vi "Actor Core.vi"(8 "error in":errorcluster, 11 "Example Actor in":refnum<class "Example Actor.lvclass">) -> (0 "error out":errorcluster, 3 "Actor out":refnum<class "Actor.lvclass">)   [LabVIEW 2023, in "Example Iterator NR Actor.lvlib" / "Example Actor.lvclass"]
doc: "(<B>Filename</B>: Actor Framework.lvlib:Actor.lvclass:Actor Core.vi)\n\nReceives messages to the actor, reacts to them, and initiates any error handling that may shut the actor down.\n\nDescendant classes may override this VI to append parallel tasks for the actor to complete while it handles messages. Overrides use the Call Parent Method node."
uses:
  Example Actor.lvclass
  C:/Program Files/National Instruments/LabVIEW 2023/vi.lib/ActorFramework/Actor/Actor.lvclass
  <vilib>/ActorFramework/Actor/Actor.lvclass
  Iterator Settings.ctl
  Abstract Iterator Actor/Active Stop Conditions.ctl
  <vilib>/ActorFramework/Message Enqueuer/Message Priority.ctl
  Abstract Iterator Actor/Stop Reason.ctl
  Iterator NR Actor/Iterator NR Actor.lvclass
  Iterator NR Actor/Iterator NR Actor.lvclass/Iterator NR Actor.ctl
  Example Actor.lvclass/Example Actor.ctl
  <vilib>/ActorFramework/Actor/Actor.lvclass/Actor.ctl
  <vilib>/ActorFramework/Message Enqueuer/Message Enqueuer.lvclass/Message Enqueuer.ctl
  Example Actor Messages/Iterate Reply Msg/Iteration Msg.lvclass
  C:/Program Files/National Instruments/LabVIEW 2023/vi.lib/ActorFramework/Message/Message.lvclass
  Abstract Iterator Actor/Iterator Settings.ctl
  <vilib>/ActorFramework/Message/Message.lvclass
  Abstract Iterator Actor Messages/Iterator Report Iterations End Msg/Iterator Report Iterations End Msg.lvclass
  Example Actor Messages/Pre Iterate Reply Msg/Pre Iteration Msg.lvclass
  Example Actor Messages/Post Iterate Reply Msg/Post Iteration Msg.lvclass
  Example Actor Messages/Update Error Msg/Update Error Msg.lvclass
  C:/Projects/Iterator Actor/Abstract Iterator Actor Messages/Iterator Report Iterations End Msg/Iterator Report Iterations End Msg.lvclass
  Iterator NR Actor/Write Auto Iteration Notification.vi
  <vilib>/ActorFramework/Message Enqueuer/Init from Existing Queue.vi
  <vilib>/ActorFramework/Message Enqueuer/Enqueue.vi
  <vilib>/ActorFramework/Stop Msg/Stop Msg.lvclass
  <vilib>/ActorFramework/Message Priority Queue/Priority Enqueue.vi
  <vilib>/ActorFramework/Message Enqueuer/Message Enqueuer.lvclass
  Abstract Iterator Actor Messages/Write Settings Msg/Write Settings Msg.lvclass
  Abstract Iterator Actor Messages/Start Iterations Msg/Start Iterations Msg.lvclass
  Abstract Iterator Actor Messages/Stop Iterations Msg/Stop Iterations Msg.lvclass
  Abstract Iterator Actor/Abstract Iterator Actor.lvclass
panel:
  out "Stop Reason":T1
  in  "Receive report":bool=TRUE
  in  "Do post-iterations":bool=TRUE
  in  "Do pre-iterations":bool=TRUE
  out "Iterator error":errorcluster
  in  "User Settings":T2={"Prepare timeout (ms)"=1000, "Iterate timeout (ms)"=1000, "Conclude timeout (ms)"=1000, "Iterate period (ms)"=1000, "Active Stop Conditions"={"Number of Iterations"=FALSE, "Time Elapsed"=FALSE, "Iteration Result"=FALSE}, "Iterations"=5, "Time before stop (ms)"=200, "Message Priority (Normal)"=enum."Normal"}
  out "Post Iterate":bool
  out "Pre Iterate":bool
  in  "exit":bool
  out "Iterate":bool
  in  "stop iterations":bool
  in  "start iterations":bool
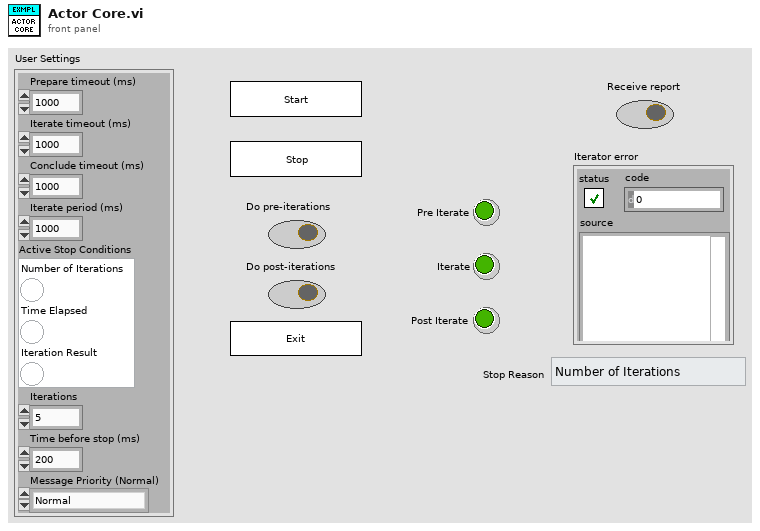
[diagram p1: front panel]
types:
  T1 = typedef "Iterator Actor.lvlib/Abstract Iterator Actor.lvclass/Stop Reason.ctl" = enum16{"Number of Iterations", "Time Elapsed", "Stopped Internally", "Stopped Externally"}
  T2 = typedef "Example Iterator NR Actor.lvlib/Example Actor.lvclass/Iterator Settings.ctl" = cluster{"Prepare timeout (ms)":i32, "Iterate timeout (ms)":i32, "Conclude timeout (ms)":i32, "Iterate period (ms)":i32, "Active Stop Conditions":T3, "Iterations":i32, "Time before stop (ms)":i32, "Message Priority (Normal)":T4}
  T3 = typedef "Iterator Actor.lvlib/Abstract Iterator Actor.lvclass/Active Stop Conditions.ctl" = cluster{"Number of Iterations":bool, "Time Elapsed":bool, "Iteration Result":bool}
  T4 = typedef "Actor Framework.lvlib/Message Enqueuer.lvclass/Message Priority.ctl" = enum16{"Low", "Normal", "High"}
  T5 = typedef "Iterator Actor.lvlib/Abstract Iterator Actor.lvclass/Iterator Settings.ctl" = cluster{"Prepare timeout (ms)":i32, "Iterate timeout (ms)":i32, "Conclude timeout (ms)":i32, "Iterate period (ms)":i32, "Number of iterations":i32, "Time before stop (ms)":i32, "Active Stop Conditions":T3, "Prepare Msg":refnum<class "Message.lvclass">, "Iterate Msg":refnum<class "Message.lvclass">, "Conclude Msg":refnum<class "Message.lvclass">, "Iterations End Report":refnum<class "Iterator Report Iterations End Msg.lvclass">, "Message Priority (Normal)":T4}
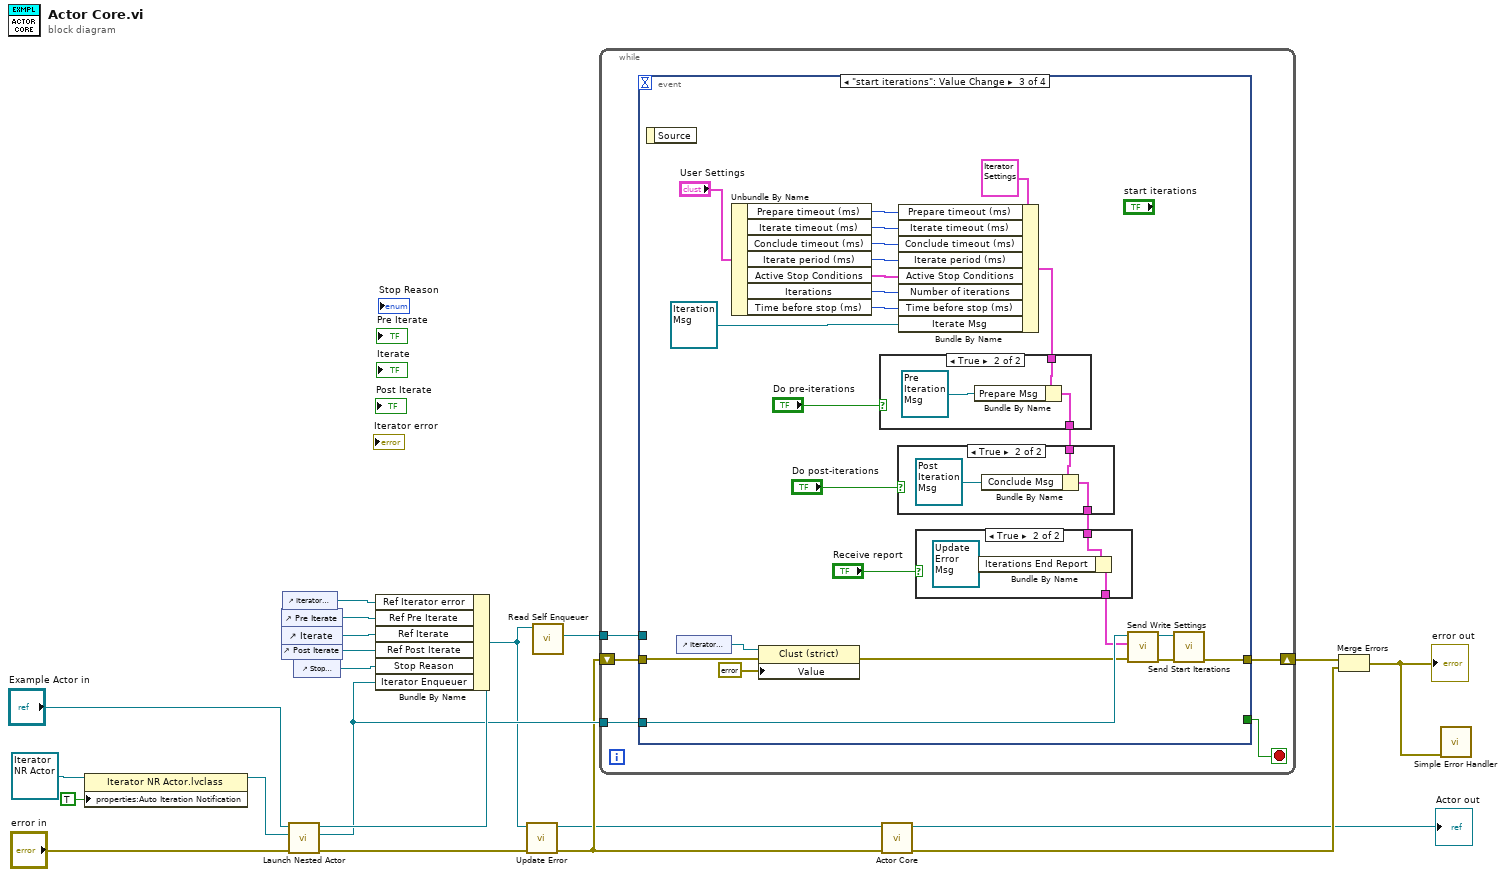
[diagram p0: block diagram]
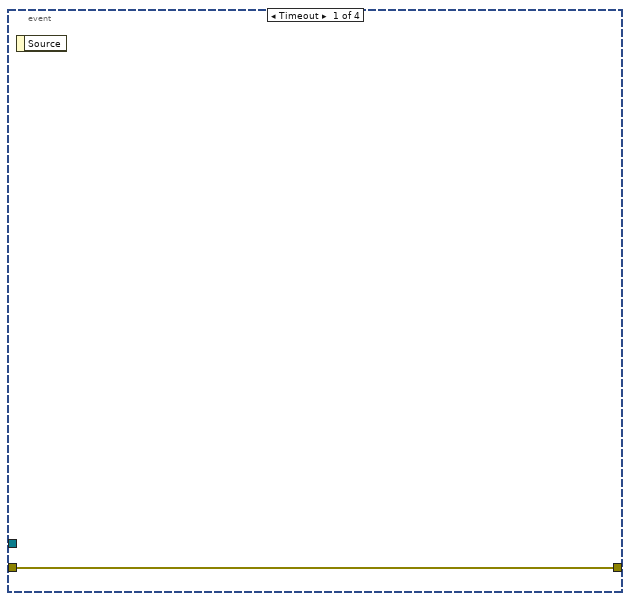
[diagram p2: hidden frame]
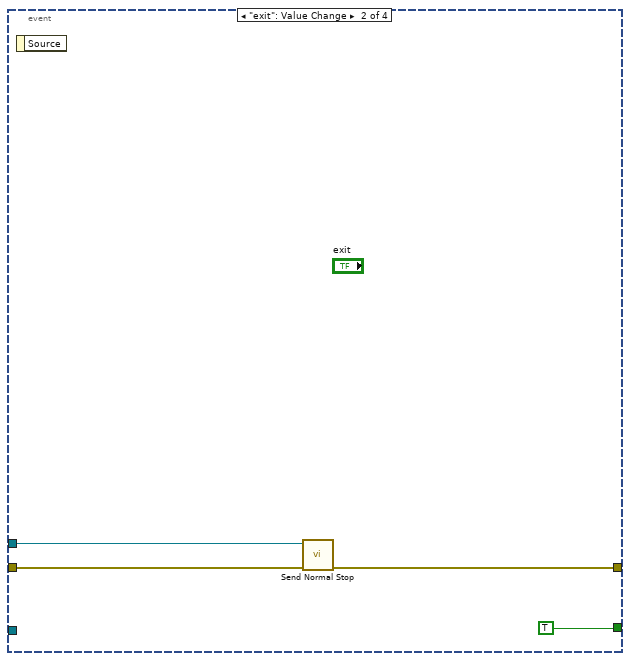
[diagram p3: hidden frame]
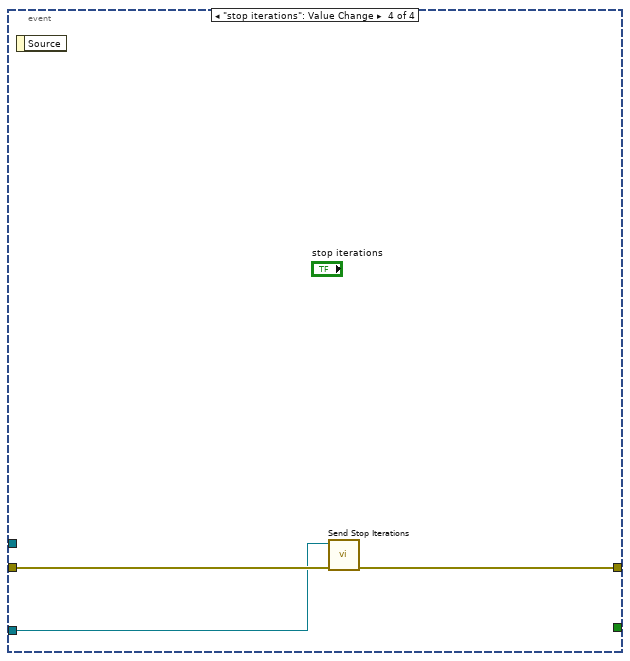
[diagram p7: hidden frame]
diagram:
  n1 = property class="Iterator NR Actor.lvclass"(reference=refnum<class "Iterator NR Actor.lvclass"> refnum ("Iterator Actor 2.lvlib:Iterator Actor 2.lvclass"), "properties:Auto Iteration Notification"=TRUE ("Auto Iteration Notification")) -> (reference out=w2:refnum<class "Iterator NR Actor.lvclass">)  [unwired: 1 in, 1 out]
  n2 = control-ref of="Pre Iterate"() -> (w17:refnum<vi>)
  n3 = control-ref of="Iterate"() -> (w16:refnum<vi>)
  n4 = control-ref of="Post Iterate"() -> (w15:refnum<vi>)
  n5 = control-ref of="Iterator error"() -> (w11:refnum<vi>)
  n6 = call <vilib>:"Launch Nested Actor.vi"("error in (no error)"="error in", "Nested Actor"=w2, "Caller Actor in"="Example Actor in") -> ("error out"=w10:errorcluster, "Nested Actor's Enqueuer"=w13:refnum<class "Message Enqueuer.lvclass">, "Caller Actor out"=w14:refnum<class "Example Actor.lvclass">)  [unwired: 6 in]
  n7 = control-ref of="Stop Reason"() -> (w6:refnum<vi>)
  n8 = Bundle By Name(cluster=w14, "Ref Iterator error"=w11, "Ref Pre Iterate"=w17, "Ref Iterate"=w16, "Ref Post Iterate"=w15, "Stop Reason"=w6, "Iterator Enqueuer"=w13) -> (w8:refnum<class "Example Actor.lvclass">)
  n9 = call "Update Error.vi"("error in (no error)"=w10, "Example Actor in"=w8) -> ("error out"=w9:errorcluster, "Example Actor out"=w7:refnum<class "Example Actor.lvclass">)  [unwired: 8 in]
  n10 = call <vilib>:"Read Self Enqueuer.vi"("Actor"=w8) -> ("Self Enqueuer"=w21:refnum<class "Message Enqueuer.lvclass">)  [unwired: 10 in]
  n11 = while {
    tunnel: w21 -> [w26]
    shift-right: [w25] -> w20
    shift-left: w9 -> [w24]
    tunnel: w13 -> [w22]
    stop <- w23 stop-if-true
    n12 = event shown="[2] \"start iterations\": Value Change" {
      selector: _ -> [_ _ _ _]
      dyn-events: _ -> [_ _ _ _]
      timeout: _ -> [_ _ _ _]
      tunnel: w26 -> [_ w31 _ _]
      tunnel: [w27 w30 w41 w70] -> w25
      tunnel: w24 -> [w27 w29 w44 w71]
      tunnel: [_ TRUE _ _] -> w23
      tunnel: w22 -> [_ _ w55 w69]
      event Timeout {
        n13 = event-data() -> ()  [unwired: 1 in, 1 out]
      }
      event "exit": Value Change {
        n14 = event-data() -> ()  [unwired: 1 in, 1 out]
        n15 = call <vilib>:"Send Normal Stop.vi"("error in (no error)"=w29, "Message Enqueuer"=w31) -> ("error out"=w30:errorcluster)  [unwired: 9 in]
      }
      event "start iterations": Value Change {
        n16 = event-data() -> ()  [unwired: 1 in, 1 out]
        n17 = control-ref of="Iterator error"() -> (w43:refnum<vi>)
        n18 = Unbundle By Name("User Settings") -> ("Prepare timeout (ms)"=w48:i32, "Iterate timeout (ms)"=w49:i32, "Conclude timeout (ms)"=w50:i32, "Iterate period (ms)"=w51:i32, "Active Stop Conditions"=w45:T3, "Iterations"=w46:i32, "Time before stop (ms)"=w47:i32)
        n19 = property class="Clust (strict)"(reference=w43, error in=w44, "Value"=errorcluster {"status"=FALSE, "code"=0, "source"=""}) -> (error out=w39:errorcluster)  [unwired: 1 out]
        n20 = Bundle By Name(cluster=T5 {"Prepare timeout (ms)"=0, "Iterate timeout (ms)"=0, "Conclude timeout (ms)"=0, "Iterate period (ms)"=0, "Number of iterations"=0, "Time before stop (ms)"=0, "Active Stop Conditions"={"Number of Iterations"=FALSE, "Time Elapsed"=FALSE, "Iteration Result"=FALSE}, "Prepare Msg"=refnum, "Iterate Msg"=refnum, "Conclude Msg"=refnum, "Iterations End Report"=refnum, "Message Priority (Normal)"=enum."Normal"} ("Iterator Settings"), "Prepare timeout (ms)"=w48, "Iterate timeout (ms)"=w49, "Conclude timeout (ms)"=w50, "Iterate period (ms)"=w51, "Active Stop Conditions"=w45, "Number of iterations"=w46, "Time before stop (ms)"=w47, "Iterate Msg"=refnum<class "Iteration Msg.lvclass"> refnum ("Example Actor.lvlib:Iterate Reply Msg.lvclass")) -> (w36:T5)
        n21 = case shown="True" "Do pre-iterations" {
          tunnel: w36 -> [w65 w68]
          tunnel: [w65 w66] -> w35
          frame False {
          }
          frame True {
            n22 = Bundle By Name(cluster=w68, "Prepare Msg"=refnum<class "Pre Iteration Msg.lvclass"> refnum ("Example Actor.lvlib:Pre Iterate Reply Msg.lvclass")) -> (w66:T5)
          }
        }
        n23 = case shown="True" "Do post-iterations" {
          tunnel: w35 -> [w61 w64]
          tunnel: [w61 w62] -> w33
          frame False {
          }
          frame True {
            n24 = Bundle By Name(cluster=w64, "Conclude Msg"=refnum<class "Post Iteration Msg.lvclass"> refnum ("Example Actor.lvlib:Post Iterate Reply Msg.lvclass")) -> (w62:T5)
          }
        }
        n25 = case shown="True" "Receive report" {
          tunnel: [w57 w60] -> w32
          tunnel: w33 -> [w57 w59]
          frame False {
          }
          frame True {
            n26 = Bundle By Name(cluster=w59, "Iterations End Report"=refnum<class "Update Error Msg.lvclass"> refnum ("Example Actor.lvlib:Update Error Msg.lvclass")) -> (w60:T5)
          }
        }
        n27 = call "Send Write Settings.vi"("error in (no error)"=w39, "Settings"=w32, "Message Enqueuer in"=w55) -> ("error out"=w56:errorcluster, "Message Enqueuer out"=w40:refnum<class "Message Enqueuer.lvclass">)  [unwired: 7 in]
        n28 = call "Send Start Iterations.vi"("error in (no error)"=w56, "Message Enqueuer in"=w40) -> ("error out"=w41:errorcluster)  [unwired: 8 in, 1 out]
      }
      event "stop iterations": Value Change {
        n29 = event-data() -> ()  [unwired: 1 in, 1 out]
        n30 = call "Send Stop Iterations.vi"("error in (no error)"=w71, "Message Enqueuer in"=w69) -> ("error out"=w70:errorcluster)  [unwired: 8 in, 1 out]
      }
    }
  }
  n31 = call-parent "Actor Core.vi"("error in"=w9, "Actor in"=w7) -> ("error out"=w19:errorcluster, "Actor out"=→"Actor out":refnum<class "Actor.lvclass">)  [unwired: 8 in]
  n32 = Merge Errors(w20, w19) -> (w12:errorcluster)
  "error out" <- w12
  n33 = call <vilib>:"Simple Error Handler.vi"("error in (no error)"=w12) -> ()  [unwired: 4 in, 5 out]
